vi "Map Loop.vi"(7 "I in":i64, 8 "error in (no error)":errorcluster, 9 "Array":refnum<vi>[](array[refnum]), 10 "MAP":refnum<vi>, 11 "Boolean in":refnum<vi>) -> (0 "error out":errorcluster, 3 "I next out":i64)   [LabVIEW 2010]
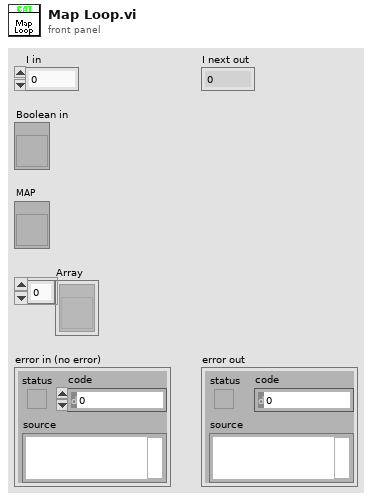
[diagram p1: front panel]
types:
  T1 = cluster{"Game Road 1":u16, "Game Road 2":u16, "Game Road 3":u16, "Game Road 4":u16, "Game Road 5":u16, "Game Road 6":u16, "Game Road 7":u16, "Game Road 8":u16, "Game Road 9":u16, "Game Road 10":u16, "Game Road 11":u16, "Game Road 12":u16, "Game Road 13":u16, "Game Road 14":u16, "Game Road 15":u16, "Game Coin 1":u16, "Game Coin 2":u16, "Game Coin 3":u16, "Game Coin 4":u16, "Game Coin 5":u16, "Game Coin 6":u16, "Game Coin 7":u16, "Game Coin 8":u16, "Game Coin 9":u16, "Game Coin 10":u16, "Game Coin 11":u16, "Game Coin 12":u16, "Game Coin 13":u16, "Game Coin 14":u16, "Game Coin 15":u16, "Game Coin 16":u16, "Game Coin 17":u16, "Game Coin 18":u16, "Game Coin 19":u16, "Game Coin 20":u16, "Game Coin 21":u16, "Game Coin 22":u16, "Game Coin 23":u16, "Game Coin 24":u16, "Game Coin 25":u16, "Game Coin 26":u16, "Game Coin 27":u16, "Game Coin 28":u16, "Game Coin 29":u16, "Game Coin 30":u16, "Game Coin 31":u16, "Game Coin 32":u16, "Game Coin 33":u16, "Game Coin 34":u16, "Game Coin 35":u16, "Game Coin 36":u16, "Game Coin 37":u16, "Game Coin 38":u16, "Game Coin 39":u16, "Game Coin 40":u16, "Game Coin 41":u16, "Game Coin 42":u16, "Game Coin 43":u16, "Game Coin 44":u16, "Game Coin 45":u16, "Game Coin 46":u16, "Game Coin 47":u16, "Game Coin 48":u16, "Game Coin 49":u16, "Game Coin 50":u16, "Game Coin 51":u16, "Game Coin 52":u16, "Game Coin 53":u16, "Game Coin 54":u16, "Game Coin 55":u16, "Game Coin 56":u16, "Game Coin 57":u16, "Game Coin 58":u16, "Game Coin 59":u16, "Game Coin 60":u16}
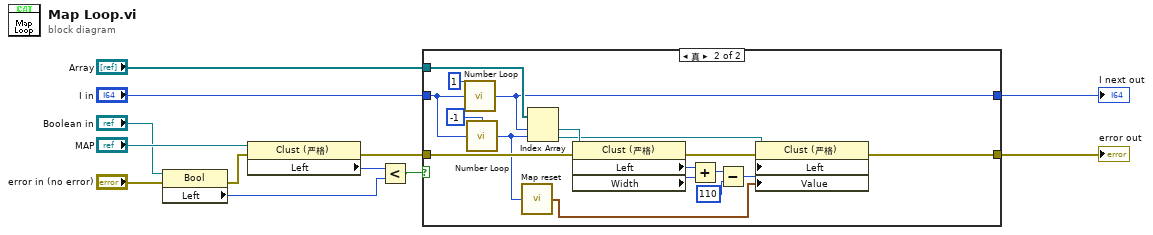
[diagram p0: block diagram]
diagram:
  n1 = property class="Bool"(reference="Boolean in", error in="error in (no error)") -> (error out=w11:errorcluster, "Left"=w9:i32)  [unwired: 1 out]
  n2 = property class="Clust (严格)"(reference="MAP", error in=w11) -> (error out=w2:errorcluster, "Left"=w7:i32)  [unwired: 1 out]
  n3 = Less?(x=w7, y=w9) -> (x < y?=w1:bool)
  n4 = case shown="真" w1 {
    tunnel: "I in" -> [w14 w18]
    tunnel: [w14 w20] -> w6
    tunnel: "Array" -> [_ w31]
    tunnel: w2 -> [w13 w26]
    tunnel: [w13 w24] -> w5
    frame False {
    }
    frame True {
      n5 = call "Number Loop.vi"("Step"=i64 1, "In"=w18) -> ("Out"=w20:i64)  [unwired: 13 in]
      n6 = call "Number Loop.vi"("Step"=i64 -1, "In"=w18) -> ("Out"=w16:i64)  [unwired: 13 in]
      n7 = call "Map reset.vi"("i"=w16) -> ("MAP"=w15:T1)  [unwired: 6 in]
      n8 = Index Array(array=w31, index #1=w20, index #2=w16) -> (element #1=w30:refnum<vi>, element #2=w29:refnum<vi>)
      n9 = property class="Clust (严格)"(reference=w30, error in=w26) -> (error out=w25:errorcluster, "Left"=w28:i32, "Width"=w27:u32)  [unwired: 1 out]
      n10 = Add(x=w28, y=w27) -> (x+y=w22:u32)
      n11 = Subtract(x=w22, y=u32 110) -> (x-y=w21:u32)
      n12 = property class="Clust (严格)"(reference=w29, error in=w25, "Left"=w21, "Value"=w15) -> (error out=w24:errorcluster)  [unwired: 1 out]
    }
  }
  "error out" <- w5
  "I next out" <- w6
